vi "Absolute Value 00.vi"(1 "x":sgl) -> (0 "abs(x)":sgl)   [LabVIEW 2015]
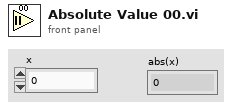
[diagram p1: front panel]
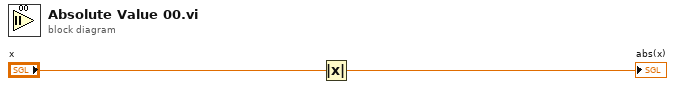
[diagram p0: block diagram]
diagram:
  n1 = Absolute Value(x="x") -> (abs(x)=→"abs(x)":sgl)
